vi "Shut_down_Hi_Tecs.vi"(4 "Client Name":string) -> ()   [LabVIEW 2018]
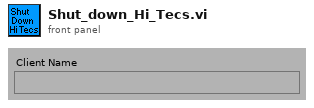
[diagram p1: front panel]
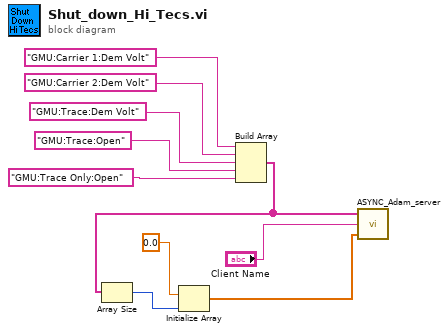
[diagram p0: block diagram]
diagram:
  n1 = Build Array("GMU:Carrier 1:Dem Volt", "GMU:Carrier 2:Dem Volt", "GMU:Trace:Dem Volt", "GMU:Trace:Open", "GMU:Trace Only:Open") -> (w5:string[])
  n2 = Array Size(array=w5) -> (size(s)=w6:i32)
  n3 = Initialize Array(0.0 ("element"), w6) -> (w3:dbl[])
  n4 = call "ASYNC_Adam_server.vi"("Values"=w3, "Client Name"="Client Name", "Channel Names"=w5) -> ()  [unwired: 3 out]
